vi "TextFit_Size Text to Fit.vi"(8 "Error":errorcluster, 9 "Size To Fit":i32, 11 "Character Array":T1[](array[typedef])) -> (0 "Error Out":errorcluster, 2 "Fit Result Out":T4, 3 "Character Array Out":T1[](array[typedef]))   [LabVIEW 2014]
doc: "Changes the Character Cluster Array's Size until the total pixel width is less than or equal to the Size to Fit input"
uses:
  Controls/Cluster/Cluster_Character Size and Priority Data.ctl
  Controls/String_Picture/String Char Normal.ctl
  Controls/Enum/ENUM_Font Size Select.ctl
  Controls/Enum/ENUM RB_Fit Result.ctl
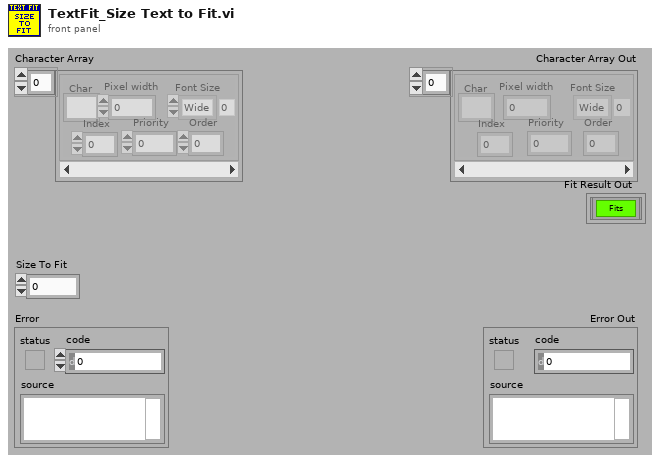
[diagram p1: front panel]
types:
  T1 = typedef "Cluster_Character Size and Priority Data.ctl" = cluster{"Char":T2, "Font Size":T3, "Pixel width":i32, "Priority":i32, "Order":i32, "Index":i32}
  T2 = typedef "String Char Normal.ctl" = string
  T3 = typedef "ENUM_Font Size Select.ctl" = enum16{"Wide", "Med", "Thin"}
  T4 = typedef "ENUM RB_Fit Result.ctl" = enum32{"Fits", "Almost Fits", "NO Fit"}
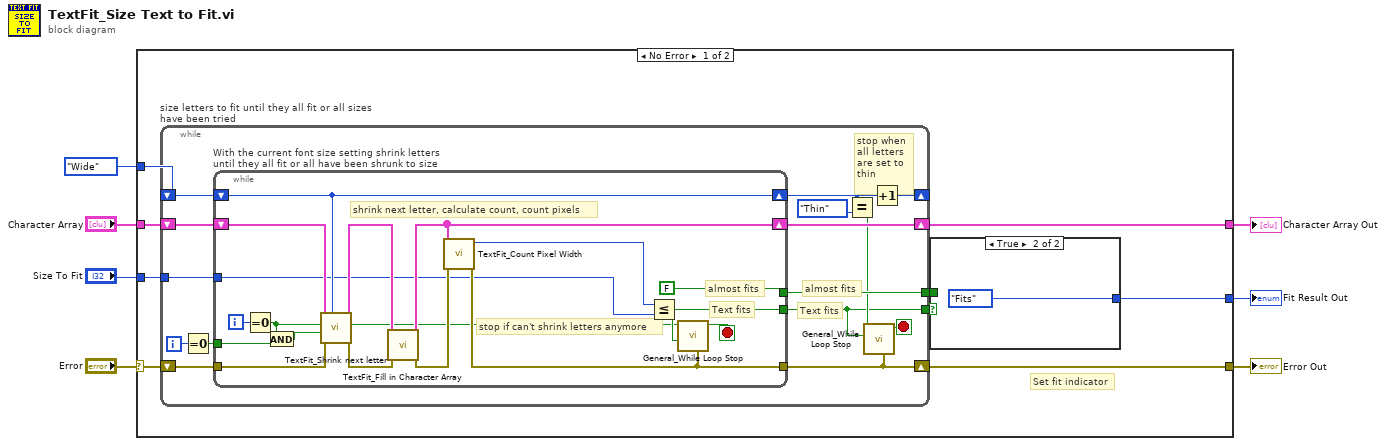
[diagram p0: block diagram]
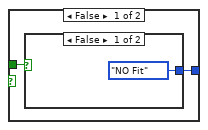
[diagram p2: hidden frame]
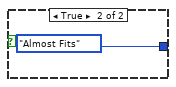
[diagram p3: hidden frame]
diagram:
  n1 = case shown="No Error" "Error" {
    selector: "Error" -> [w11 w55]
    tunnel: "Size To Fit" -> [w10 _]
    tunnel: [w9 w55] -> w6
    tunnel: [w15 _] -> w5
    tunnel: ENUM_Font_Size_Select."Wide" ("Font Size Select In") -> [w13 _]
    tunnel: "Character Array" -> [w12 w56]
    tunnel: [w8 w56] -> w1
    frame No Error {
      # "Set fit indicator"
      n2 = while "size letters to fit until they all fit or all sizes have been tried" {
        shift-right: [w31] -> w9
        shift-left: w11 -> [w34]
        tunnel: [w23] -> w14
        tunnel: [w36] -> w16
        shift-right: [w28] -> _
        shift-left: w13 -> [w33]
        shift-right: [w32] -> w8
        shift-left: w12 -> [w35]
        tunnel: w10 -> [w22]
        i -> [w27]
        stop <- w25 stop-if-true
        # "almost fits"
        # "stop when\nall letters\nare set to \nthin"
        # "Text fits"
        n3 = Equal To 0?(x=w27) -> (x = 0?=w26:bool)
        n4 = while "With the current font size setting shrink letters until they all fit or all have been shrunk to size" {
          tunnel: [w54] -> w31
          tunnel: [w53] -> w23
          tunnel: [FALSE] -> w36
          tunnel: w34 -> [w51]
          shift-right: [w45] -> w29
          shift-left: w33 -> [w45]
          tunnel: w26 -> [w43]
          shift-right: [w47] -> w32
          shift-left: w35 -> [w52]
          tunnel: w22 -> [w38]
          i -> [w44]
          stop <- w41 stop-if-true
          # "almost fits"
          # "shrink next letter, calculate count, count pixels"
          # "stop if can't shrink letters anymore"
          # "Text fits"
          n5 = Equal To 0?(x=w44) -> (x = 0?=w40:bool)
          n6 = And(x=w40, y=w43) -> (x .and. y?=w39:bool)
          n7 = call "TextFit_Shrink next letter.vi"("Font Size"=w45, "Error"=w51, "Do Not Shrink"=w39, "Reset Prioity"=w40, "Character Array"=w52) -> ("Error Out"=w50:errorcluster, "All Items Shrunk Out"=w46:bool, "Character Array Out"=w48:T1[])  [unwired: 4 in]
          n8 = call "TextFit_Fill in Character Array.vi"("Error"=w50, "Character Array"=w48) -> ("Error Out"=w49:errorcluster, "Character Array Out"=w47:T1[])  [unwired: 8 in]
          n9 = call "TextFit_Count Pixel Width.vi"("Error"=w49, "Counter Array"=w47) -> ("Error Out"=w54:errorcluster, "Pixel Width Out"=w42:i32)  [unwired: 8 in]
          n10 = Less Or Equal?(x=w42, y=w38) -> (x <= y?=w53:bool)
          n11 = call "General_While Loop Stop.vi"("Error In"=w54, "Stop 3 In"=w53, "Stop 1 In"=w46) -> ("Stop Out1"=w41:bool)  [unwired: 4 in, 3 out]
        }
        n12 = Equal?(x=w29, y=ENUM_Font_Size_Select."Thin") -> (x = y?=w24:bool)
        n13 = call "General_While Loop Stop.vi"("Error In"=w31, "Stop 2 In"=w23, "Stop 1 In"=w24) -> ("Stop Out1"=w25:bool)  [unwired: 4 in, 3 out]
        n14 = Increment(x=w29) -> (x+1=w28:T3)
      }
      n15 = case shown="True" w14 {
        tunnel: [w17 ENUM_RB_Fit_Result."Fits" ("Fit Result")] -> w15
        tunnel: w16 -> [w18 _]
        frame False {
          n16 = case shown="False" w18 {
            tunnel: [ENUM_RB_Fit_Result."NO Fit" ("Fit Result") ENUM_RB_Fit_Result."Almost Fits" ("Fit Result")] -> w17
            frame False {
            }
            frame True {
            }
          }
        }
        frame True {
        }
      }
    }
    frame Error {
    }
  }
  "Error Out" <- w6
  "Character Array Out" <- w1
  "Fit Result Out" <- w5
